vi "CAN Data  Convert String To Hex.vi"(11 "String":string) -> (2 "number":u32[](array[numeric]), 3 "appended array":string[](array[string]))   [LabVIEW 2015]
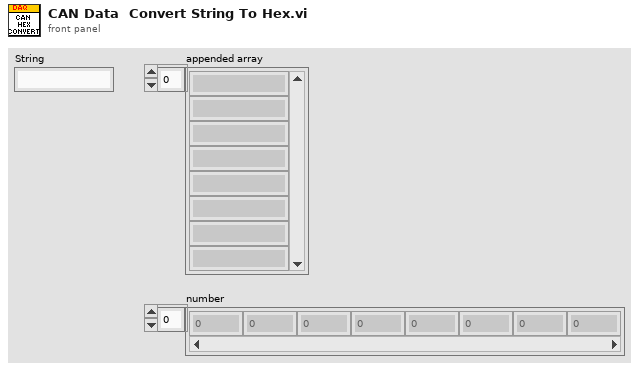
[diagram p1: front panel]
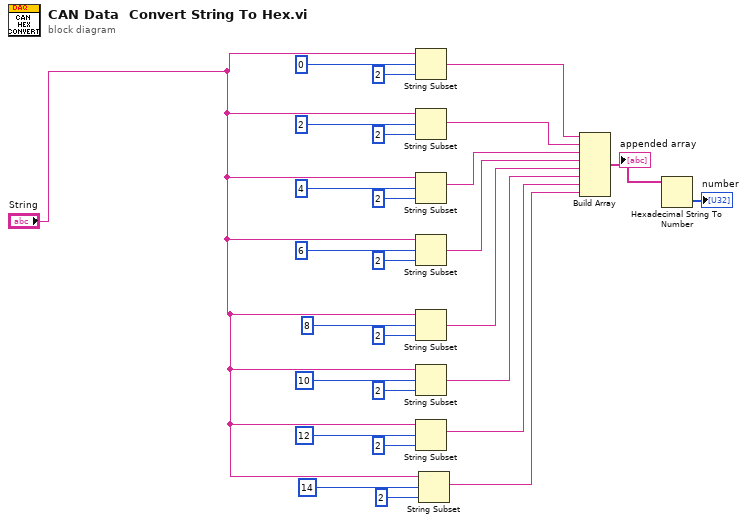
[diagram p0: block diagram]
diagram:
  n1 = String Subset(string="String", offset (0)=0, length (rest)=2 ("length (rest)")) -> (substring=w15:string)
  n2 = String Subset(string="String", offset (0)=2, length (rest)=2 ("length (rest)")) -> (substring=w16:string)
  n3 = String Subset(string="String", offset (0)=4, length (rest)=2 ("length (rest)")) -> (substring=w17:string)
  n4 = String Subset(string="String", offset (0)=6, length (rest)=2 ("length (rest)")) -> (substring=w18:string)
  n5 = String Subset(string="String", offset (0)=8, length (rest)=2 ("length (rest)")) -> (substring=w19:string)
  n6 = String Subset(string="String", offset (0)=10, length (rest)=2 ("length (rest)")) -> (substring=w20:string)
  n7 = String Subset(string="String", offset (0)=12, length (rest)=2 ("length (rest)")) -> (substring=w21:string)
  n8 = String Subset(string="String", offset (0)=14, length (rest)=2 ("length (rest)")) -> (substring=w25:string)
  n9 = Build Array(w15, w16, w17, w18, w19, w20, w21, w25) -> (w26:string[])
  "appended array" <- w26
  n10 = Hexadecimal String To Number(string=w26) -> (number=→"number":u32[])  [unwired: 2 in, 1 out]
